vi "Construct Create ZIP Step.vi"(5 "Create ZIP Step in":refnum<class "Create ZIP Step.lvclass">, 8 "error in (no error)":errorcluster, 11 "ZIP Model":T1) -> (0 "error out":errorcluster, 3 "Create ZIP Step":refnum<class "Create ZIP Step.lvclass">)   [LabVIEW 2019, in "ZIP.lvlib" / "Create ZIP Step.lvclass"]
uses:
  Create ZIP Step.lvclass
  ZIP Model.ctl
  Create ZIP Step.lvclass/Create ZIP Step.ctl
  ZIP.lvlib
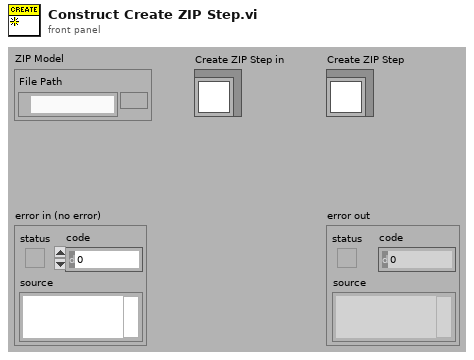
[diagram p1: front panel]
types:
  T1 = typedef "ZIP.lvlib/ZIP Model.ctl" = cluster{"File Path":path}
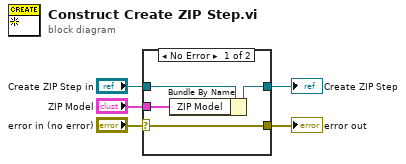
[diagram p0: block diagram]
diagram:
  n1 = case shown="No Error" "error in (no error)" {
    selector: "error in (no error)" -> [w9 w11]
    tunnel: [w9 w11] -> w4
    tunnel: [w7 w10] -> w2
    tunnel: "Create ZIP Step in" -> [w8 w10]
    tunnel: "ZIP Model" -> [w6 _]
    frame No Error {
      n2 = Bundle By Name(cluster=w8, "ZIP Model"=w6) -> (w7:refnum<class "Create ZIP Step.lvclass">)
    }
    frame Error {
    }
  }
  "error out" <- w4
  "Create ZIP Step" <- w2
